vi "12.-Leer un Archivo y Pasarlo a un String.vi"() -> ()   [LabVIEW 2020]
panel:
  out "error out":errorcluster
  out "text":string
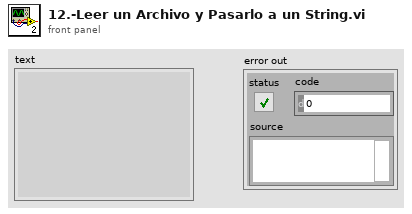
[diagram p1: front panel]
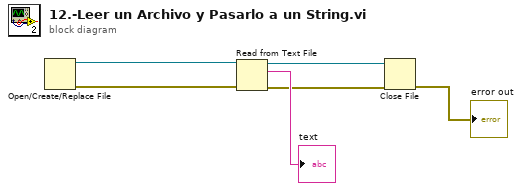
[diagram p0: block diagram]
diagram:
  n1 = Open/Create/Replace File() -> (refnum out=w6:refnum<file>, error out=w5:errorcluster)  [unwired: 6 in, 1 out]
  n2 = Read from Text File(file (use dialog)=w6, error in=w5) -> (refnum out=w3:refnum<file>, text=→"text":string, error out=w2:errorcluster)  [unwired: 2 in, 1 out]
  n3 = Close File(refnum=w3, error in=w2) -> (error out=→"error out":errorcluster)  [unwired: 1 out]
